vi "Write Read Wait.vi"(0 "Valve Channel":i32, 5 "Open/ Close Valve":bool, 7 "Sensor Channel":i32, 9 "Desired Sensor Value":bool, 11 "Initial State":bool[](array[boolean]), 12 "error in (no error)":errorcluster) -> (4 "FinalState":bool[](array[boolean]), 14 "error out":errorcluster)   [LabVIEW 2016]
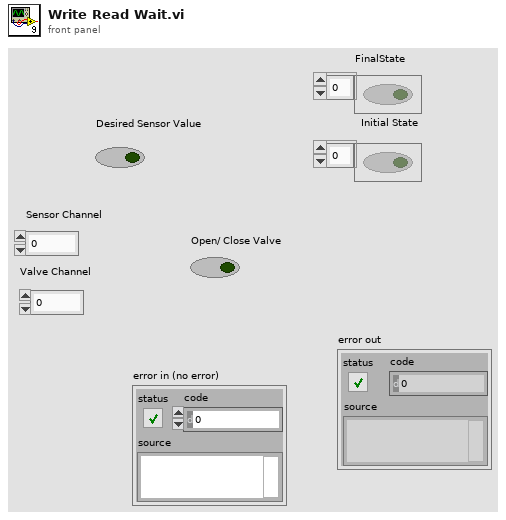
[diagram p1: front panel]
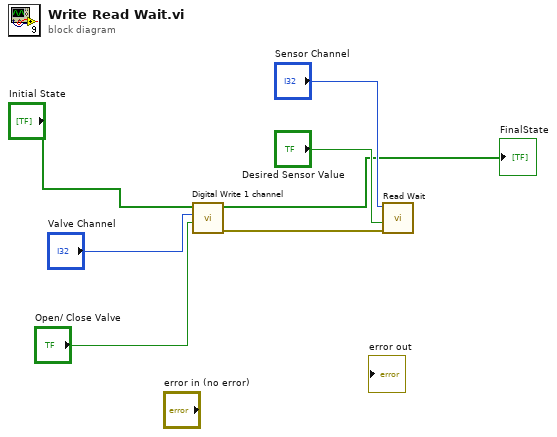
[diagram p0: block diagram]
diagram:
  n1 = call "Digital Write 1 channel.vi"("On/Off"="Open/ Close Valve", "Channel"="Valve Channel", "Initial State"="Initial State") -> ("error out"=w4:errorcluster, "FinalState"=→"FinalState":bool[])  [unwired: 7 in]
  n2 = call "Read Wait.vi"("Sensor Channel"="Sensor Channel", "Desired Value"="Desired Sensor Value", "error in (no error)"=w4) -> ()  [unwired: 7 in, 1 out]
